vi "Lab7_Swept Sine Data Recoding v3 (1).vi"() -> ()   [LabVIEW 2016]
uses:
  <vilib>/Utility/error.llb/DialogType.ctl
  <vilib>/DAQmx/write.llb/DAQmx Write (Analog 1D Wfm NChan NSamp).vi
  <vilib>/express/express analysis/Spectral/Block/exnSpectralBlock spectral measurements RMS poly.vi
  <vilib>/express/express analysis/Spectral/Block/exnSpectralBlock spectral measurements RMS DDT.vi
  <vilib>/Utility/file.llb/Write Delimited Spreadsheet (string).vi
  <vilib>/measure/matone.llb/Extract Single Tone Information N Chan.vi
  <vilib>/Utility/file.llb/Write Delimited Spreadsheet (DBL).vi
  <vilib>/DAQmx/create/channels.llb/DAQmx Create Channel (AO-Voltage-Basic).vi
  <vilib>/DAQmx/configure/timing.llb/DAQmx Timing (Sample Clock).vi
  <vilib>/DAQmx/miscellaneous.llb/DAQmx Fill In Error Info.vi
  <vilib>/express/express analysis/Spectral/XNode/ExpressSpectralMeasurementsBlockNode.xnode
  <vilib>/measure/NI_MAPro.lvlib
  <resource>/objmgr/daqmx.rc
  <vilib>/measure/NI_MABase.lvlib
panel:
  in  "Analog Out Channel":tag="cDAQ1Mod2/ao0"
  in  "stop (F) 2":bool caption="stop (F)"
  out "Waveform Graph":waveform(dbl)[](graph)=[{"t0"=timestamp(0 s since 1904-01-01), "dt"=0.001, "Y"=[]}]
  in  "Frequency":dbl
  in  "Amplitude":dbl format="%#_13g"
  out "Actual Sample Rate":dbl=1000.0 format="%0.2f"
  in  "filename (end in .csv)":string
  in  "Dwell Time (s)":i16=500
  in  "Sweep":bool
  in  "End Freq":i16=10 caption="Frequency"
  in  "Start Freq":i16=10 caption="Frequency"
  out "Mean":dbl[](array[numeric])
  out "FFT Amplitude":dynamicdata(graph)
  out "Raw In":dynamicdata(graph) caption="Raw"
  in  "stop (F)":bool
  # "Manual Output Control"
  # "Automatic Swept Sine"
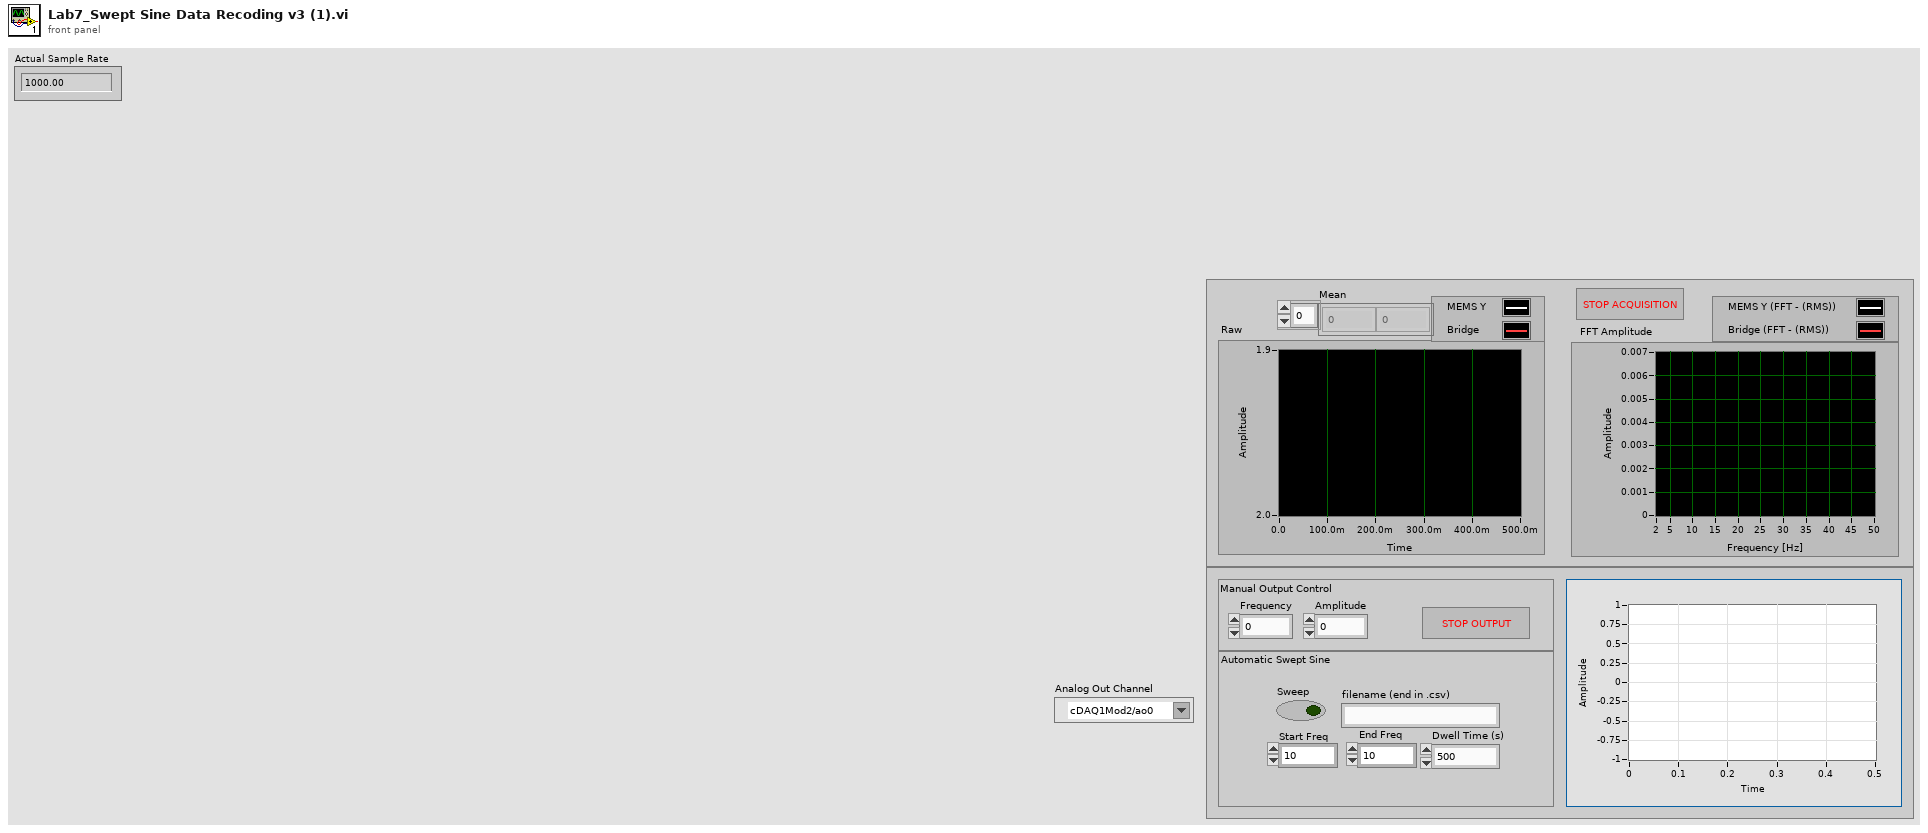
[diagram p1: front panel]
types:
  T1 = cluster{"Waveform Type":u16, "Amplitude":dbl, "Frequency":dbl}
  T2 = typedef "DialogType.ctl" = u16
  T3 = cluster{"averaging mode":u16, "weighting mode":u16, "number of averages":u32}
  T4 = cluster{"dB On (F)":bool, "unwrap phase (F)":bool, "convert to degree (F)":bool}
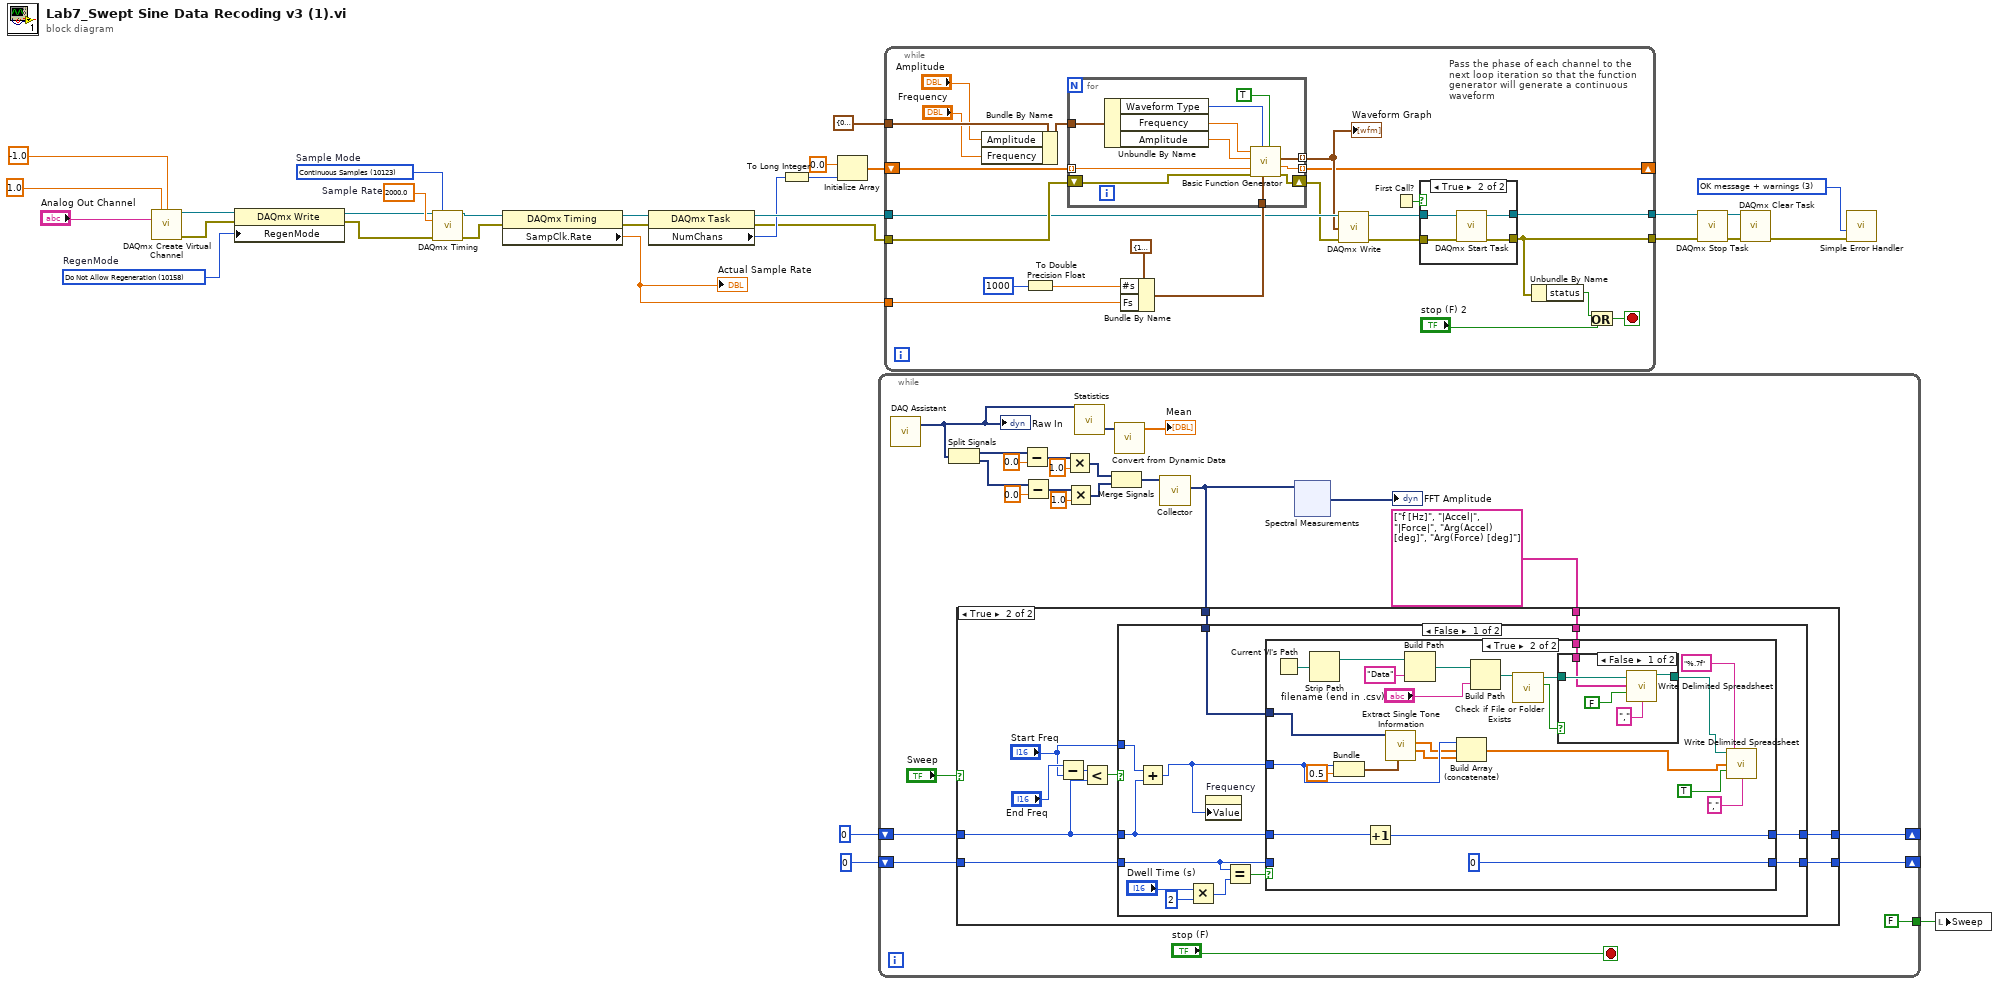
[diagram p0: block diagram]
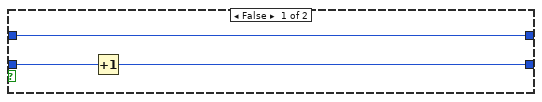
[diagram p4: hidden frame]
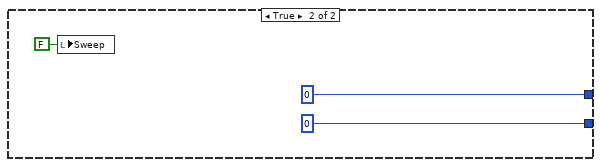
[diagram p6: hidden frame]
diagram:
  w25 = 2000.0  # Sample Rate
  w12 = T2 3 items=["no dialog", "OK message", "continue or stop message", "OK message + warnings", "continue/stop + warnings"] ("type of dialog (OK msg:1)")
  w19 = 10158 items=["Allow Regeneration"=10097, "Do Not Allow Regeneration"=10158]  # RegenMode
  w28 = 10123 items=["Finite Samples"=10178, "Continuous Samples"=10123, "Hardware Timed Single Point"=12522]  # Sample Mode
  n1 = call-poly <vilib>:"DAQmx Create Virtual Channel.vi"("maximum value"=1.0 ("Max Voltage"), "minimum value"=-1.0 ("Min Voltage"), "physical channels"="Analog Out Channel") -> ("task out"=w21:refnum<k21>, "error out"=w20:errorcluster)  [unwired: 11 in]
  n2 = property class="DAQmx Write"(reference=w21, error in=w20, "RegenMode"=w19) -> (reference out=w17:refnum<k21>, error out=w18:errorcluster)
  n3 = call-poly <vilib>:"DAQmx Timing.vi"("task/channels in"=w17, "sample mode"=w28, "rate"=w25, "error in"=w18) -> ("task out"=w4:refnum<k21>, "error out"=w3:errorcluster)  [unwired: 10 in]
  n4 = property class="DAQmx Timing"(reference=w4, error in=w3) -> (reference out=w8:refnum<k21>, error out=w7:errorcluster, "SampClk.Rate"=w22:dbl)
  "Actual Sample Rate" <- w22
  n5 = property class="DAQmx Task"(reference=w8, error in=w7) -> (reference out=w9:refnum<k21>, error out=w1:errorcluster, "NumChans"=w6:u32)
  n6 = To Long Integer(number=w6) -> (32bit integer=w5:i32)
  n7 = Initialize Array(0.0 ("element"), w5) -> (w10:dbl[])
  n8 = while {
    shift-right: [w41] -> _
    shift-left: i16 0 ("End") -> [w42]
    shift-right: [w40] -> _
    shift-left: i16 0 ("End") -> [w37]
    tunnel: [FALSE ("Sweep")] -> w29
    stop <- "stop (F)" stop-if-true
    n9 = call "DAQ Assistant"() -> ("data"=w32:dynamicdata)  [unwired: 16 in, 3 out]
    "Raw In" <- w32
    n10 = Split Signals(w32) -> (w49:dynamicdata, w48:dynamicdata)  [unwired: 2 in]
    n11 = Subtract(x=w49, y=0.0) -> (x-y=w55:dynamicdata)
    n12 = Subtract(x=w48, y=0.0) -> (x-y=w52:dynamicdata)
    n13 = Multiply(x=w55, y=1.0) -> (x*y=w47:dynamicdata)
    n14 = Multiply(x=w52, y=1.0) -> (x*y=w46:dynamicdata)
    n15 = call "Statistics"("Signals"=w32) -> ("Arithmetic Mean"=w44:dynamicdata)  [unwired: 25 in, 1 out]
    n16 = Merge Signals(w47, w46) -> (w45:dynamicdata)
    n17 = call "Convert from Dynamic Data"("Dynamic Data Type"=w44) -> ("Array"=→"Mean":dbl[])  [unwired: 3 in]
    n18 = call "Collector"("Signals"=w45) -> ("Collected Signals"=w39:dynamicdata)  [unwired: 9 in, 1 out]
    n19 = case shown="True" "Sweep" {
      tunnel: w42 -> [w56 w67]
      tunnel: [w56 w66] -> w41
      tunnel: [w57 w65] -> w40
      tunnel: w39 -> [_ w64]
      tunnel: w37 -> [w57 w62]
      tunnel: string[] ["f [Hz]", "|Accel|", "|Force|", "Arg(Accel) [deg]", "Arg(Force) [deg]"] ("1D data") -> [_ w58]
      frame False {
      }
      frame True {
        n20 = Subtract(x="End Freq", y="Start Freq") -> (x-y=w63:i16)
        n21 = Less?(x=w63, y=w62) -> (x < y?=w61:bool)
        n22 = case shown="False" w61 {
          tunnel: w67 -> [w78 _]
          tunnel: [w77 i16 0] -> w66
          tunnel: [w76 i16 0 ("End")] -> w65
          tunnel: w64 -> [w75 _]
          tunnel: w62 -> [w74 _]
          tunnel: "Start Freq" -> [w73 _]
          tunnel: w58 -> [w69 _]
          frame False {
            n23 = Add(x=w73, y=w74) -> (x+y=w68:i16)
            n24 = Multiply(x="Dwell Time (s)", y=i16 2) -> (x*y=w72:i16)
            n25 = property on="Frequency" class="DigNum (strict)"("Value"=w68) -> ()  [unwired: 2 in, 2 out]
            n26 = Equal?(x=w78, y=w72) -> (x = y?=w79:bool)
            n27 = case shown="True" w79 {
              tunnel: w78 -> [w82 _]
              tunnel: [w81 i16 0] -> w77
              tunnel: w74 -> [w80 w98]
              tunnel: [w80 w104] -> w76
              tunnel: w75 -> [_ w94]
              tunnel: w68 -> [_ w97]
              tunnel: w69 -> [_ w88]
              frame False {
                n28 = Increment(x=w82) -> (x+1=w81:i16)
              }
              frame True {
                n29 = Current VI's Path() -> (path=w100:path)
                n30 = Strip Path(path=w100) -> (stripped path=w99:path)  [unwired: 1 out]
                n31 = Bundle(w97, "search (+/- % of Fsampl.)"=0.5) -> (w95:cluster{i16, "search (+/- % of Fsampl.)":dbl})  [unwired: 1 in]
                n32 = Increment(x=w98) -> (x+1=w104:i16)
                n33 = call-poly <vilib>:"Extract Single Tone Information.vi"("advanced search"=w95, "time signals in"=w94) -> ("detected phases (deg)"=w92:dbl[], "detected amplitudes"=w93:dbl[])  [unwired: 4 in, 4 out]
                n34 = Build Path(base path=w99, name or relative path="Data") -> (appended path=w102:path)
                n35 = Build Array (concatenate)(w97, w93, w92) -> (w85:dbl[])
                n36 = Build Path(base path=w102, name or relative path="filename (end in .csv)") -> (appended path=w91:path)
                n37 = call <vilib>:"Check if File or Folder Exists.vi"("path"=w91) -> ("file or folder exists?"=w90:bool, "dup path"=w89:path)  [unwired: 8 in, 1 out]
                n38 = case shown="False" w90 {
                  tunnel: w89 -> [w110 w111]
                  tunnel: [w109 w111] -> w86
                  tunnel: w88 -> [w107 _]
                  frame False {
                    n39 = call-poly <vilib>:"Write Delimited Spreadsheet.vi"("file path (dialog if empty)"=w110, "1D data"=w107, "append to file? (new file:F)"=FALSE, "delimiter (\\t)"="," ("delimiter (\\t)")) -> ("new file path (Not A Path if cancelled)"=w109:path)  [unwired: 10 in, 1 out]
                  }
                  frame True {
                  }
                }
                n40 = call-poly <vilib>:"Write Delimited Spreadsheet.vi"("file path (dialog if empty)"=w86, "format (%.3f)"="%.7f", "1D data"=w85, "append to file? (new file:F)"=TRUE, "delimiter (\\t)"="," ("delimiter (\\t)")) -> ()  [unwired: 9 in, 2 out]
              }
            }
          }
          frame True {
            n41 = local write "Sweep"(FALSE ("Sweep")) -> ()
          }
        }
      }
    }
    n42 = xnode "Spectral Measurements"("Signals"=w39) -> ("FFT - (RMS)"=→"FFT Amplitude":dynamicdata)  [unwired: 1 in, 2 out]
  }
  n43 = while {
    tunnel: w1 -> [w147]
    tunnel: w22 -> [w145]
    tunnel: w9 -> [w143]
    tunnel: [w135] -> w14
    tunnel: [w134] -> w13
    shift-right: [w131] -> _
    shift-left: w10 -> [w130]
    tunnel: T1 {"Waveform Type"=0, "Amplitude"=1.0, "Frequency"=10.5} ("Cluster") -> [w129]
    stop <- w133 stop-if-true
    # "Pass the phase of each channel to the next loop iteration so that the function generator will generate a continuous waveform"
    n44 = Bundle By Name(cluster=w129, "Amplitude"="Amplitude", "Frequency"="Frequency") -> (w128:T1)
    n45 = To Double Precision Float(number=1000 ("Number of Samples")) -> (double precision float=w138:dbl)
    n46 = Bundle By Name(cluster=cluster{"Fs":dbl, "#s":dbl} {"Fs"=1000.0, "#s"=1000.0} ("sampling info"), "#s"=w138, "Fs"=w145) -> (w144:cluster{"Fs":dbl, "#s":dbl})
    n47 = for {
      tunnel: w144 -> [w163]
      tunnel: w128 -> [w161]
      tunnel: [w157] -> w139 mode=indexing
      tunnel: [w156] -> w131 mode=indexing
      tunnel: w130 -> [w154] mode=indexing
      shift-right: [w162] -> w140
      shift-left: w147 -> [w164]
      n48 = Unbundle By Name(w161) -> ("Waveform Type"=w160:u16, "Frequency"=w159:dbl, "Amplitude"=w158:dbl)
      n49 = call <vilib>:"Basic Function Generator.vi"("reset signal"=TRUE, "sampling info"=w163, "signal type"=w160, "error in (no error)"=w164, "phase"=w154, "amplitude"=w158, "frequency"=w159) -> ("error out"=w162:errorcluster, "phase out"=w156:dbl, "signal out"=w157:waveform(dbl))  [unwired: 2 in]
    }
    "Waveform Graph" <- w139
    n50 = call-poly <vilib>:"DAQmx Write.vi"("task/channels in"=w143, "data"=w139, "error in"=w140) -> ("task out"=w142:refnum<k21>, "error out"=w141:errorcluster)  [unwired: 10 in, 1 out]
    n51 = First Call?() -> (First Call?: T/F=w136:bool)
    n52 = case shown="True" w136 {
      tunnel: w142 -> [w148 w153]
      tunnel: w141 -> [w149 w152]
      tunnel: [w148 w151] -> w135
      tunnel: [w149 w150] -> w134
      frame False {
      }
      frame True {
        n53 = call <vilib>:"DAQmx Start Task.vi"("task/channels in"=w153, "error in"=w152) -> ("task out"=w151:refnum<k21>, "error out"=w150:errorcluster)  [unwired: 12 in]
      }
    }
    n54 = Unbundle By Name(w134) -> ("status"=w132:bool)
    n55 = Or(x=w132, y="stop (F) 2") -> (x .or. y?=w133:bool)
  }
  n56 = call <vilib>:"DAQmx Stop Task.vi"("task/channels in"=w14, "error in"=w13) -> ("task out"=w16:refnum<k21>, "error out"=w15:errorcluster)  [unwired: 12 in]
  n57 = call <vilib>:"DAQmx Clear Task.vi"("task in"=w16, "error in"=w15) -> ("error out"=w27:errorcluster)  [unwired: 13 in]
  n58 = call <vilib>:"Simple Error Handler.vi"("type of dialog (OK msg:1)"=w12, "error in (no error)"=w27) -> ()  [unwired: 3 in, 5 out]
  n59 = local write "Sweep"(w29) -> ()
